vi "Load.vi"(8 "error in (no error)":errorcluster, 10 "JSON":string, 11 "TopLevel in":refnum<class "TopLevel.lvclass">) -> (0 "error out":errorcluster, 3 "TopLevel out":refnum<class "TopLevel.lvclass">)   [LabVIEW 2019, in "TopLevel.lvlib" / "TopLevel.lvclass"]
uses:
  TopLevel.lvclass
  Vision/Vision Messages/Load Msg/Load Msg.lvclass/Load Msg.ctl
  <vilib>/ActorFramework/Message Enqueuer/Message Enqueuer.lvclass/Message Enqueuer.ctl
  <vilib>/JDP Science/JSONtext/String Subset.vi
  <vilib>/ActorFramework/Message Enqueuer/Enqueue.vi
  Vision/Vision Messages/Load Msg/Load Msg.lvclass
  C:/Program Files/National Instruments/LabVIEW 2019/vi.lib/ActorFramework/Message/Message.lvclass
  <vilib>/JDP Science/JSONtext/Parsing/Parse Full Path or Item Name.vi
  <vilib>/JDP Science/JSONtext/Next JSON Value.vi
  <vilib>/JDP Science/JSONtext/support/Error Cluster From Code.vi
  <vilib>/JDP Science/JSONtext/Offset/Find Item Locations by Path.vi
  <vilib>/ActorFramework/Message Priority Queue/Priority Enqueue.vi
  <vilib>/JDP Science/JSONtext/JSONtext.lvlib
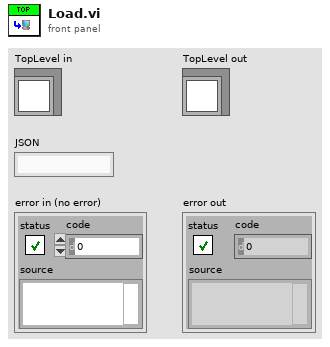
[diagram p1: front panel]
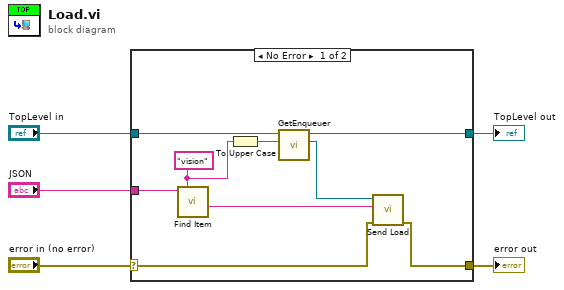
[diagram p0: block diagram]
diagram:
  n1 = case shown="No Error" "error in (no error)" {
    selector: "error in (no error)" -> [w7 w16]
    tunnel: [w6 w16] -> w4
    tunnel: [w10 w15] -> w2
    tunnel: "TopLevel in" -> [w13 w15]
    tunnel: "JSON" -> [w14 _]
    frame No Error {
      w12 = "vision" ("$Path or Item Name")
      n2 = call <vilib>:"Find Item.vi"("$Path or Item Name"=w12, "JSON"=w14) -> ("<JSON>"=w8:string)  [unwired: 6 in, 3 out]
      n3 = To Upper Case(1:w12) -> (0:w11:string)
      n4 = call "GetEnqueuer.vi"("Actor Name"=w11, "TopLevel in"=w13) -> ("Enqueuer"=w9:refnum<class "Message Enqueuer.lvclass">, "TopLevel out"=w10:refnum<class "TopLevel.lvclass">)  [unwired: 7 in, 1 out]
      n5 = call "Send Load.vi"("error in (no error)"=w7, "JSON"=w8, "Message Enqueuer"=w9) -> ("error out"=w6:errorcluster)  [unwired: 7 in, 1 out]
    }
    frame Error {
    }
  }
  "error out" <- w4
  "TopLevel out" <- w2
